vi "Engine Simulation Initialization VI.vi"(8 "error in (no error)":errorcluster, 10 "Custom XML":string, 11 "Device Item Ref in":T1 format="%.0x") -> (0 "error out":errorcluster, 3 "Device Item Ref out":T1 format="%.0x")   [LabVIEW 2011, in "Engine Sim System Explorer.lvlib"]
uses:
  Engine Sim System Explorer.lvlib
  <vilib>/NI Veristand/Custom Device API/Custom Device Item Ref.ctl
  <vilib>/NI Veristand/Custom Device API/Custom Device Loop Type.ctl
  Shared/Engine Simulation Global.vi
  <vilib>/NI Veristand/Custom Device API/Set Item Property (String).vi
  <vilib>/NI Veristand/Custom Device API/Set Item Property (Boolean).vi
  <vilib>/NI Veristand/Custom Device API/Custom Device API.lvlib
  Engine Simulation Shared.lvlib
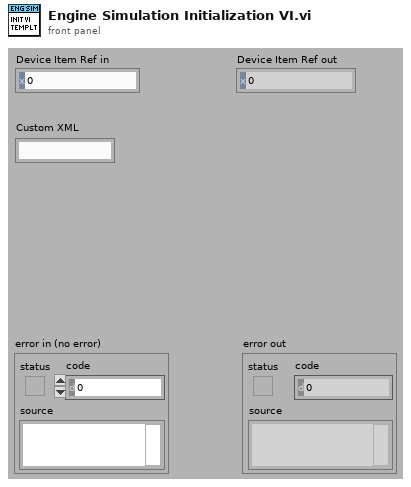
[diagram p1: front panel]
types:
  T1 = typedef "Custom Device API.lvlib/Custom Device Item Ref.ctl" = u64
  T2 = typedef "Custom Device API.lvlib/Custom Device Loop Type.ctl" = enum32{"While Loop", "Timed Loop"}
  T3 = typedef "Engine Sim System Explorer.lvlib/EngineSimComps.ctl" = cluster{"APU Component":T4, "NTeeth Components":T5[], "FullyCustom Components":T6[], "ECUEvent Components":T9[], "DataReplay Components":T10[]}
  T4 = typedef "Engine Sim System Explorer.lvlib/APUComp.ctl" = cluster{"Crank Angle":bool, "Cycle Angle":bool, "Reset":bool}
  T5 = typedef "Engine Sim System Explorer.lvlib/NTeethComp.ctl" = cluster{"Name":string, "TDC Offset":bool}
  T6 = typedef "Engine Sim System Explorer.lvlib/FullyCustomComp.ctl" = cluster{"Name":string, "Comm Mode":T7, "Profiles":T8[]}
  T7 = typedef "Engine Simulation Shared.lvlib/FullyCustomCommMode.ctl" = enum16{"DMA FIFO", "FP Data Transfer"}
  T8 = typedef "Engine Sim System Explorer.lvlib/FullyCustomProfilesComp.ctl" = cluster{"Name":string, "Offset?":bool}
  T9 = typedef "Engine Sim System Explorer.lvlib/ECUEventComp.ctl" = cluster{"Name":string, "Time Duration":bool, "Start Angle":bool, "End Angle":bool, "Angle Duration":bool}
  T10 = typedef "Engine Sim System Explorer.lvlib/DataReplayLoopComp.ctl" = cluster{"Name":string, "DataReplays":T11[]}
  T11 = typedef "Engine Sim System Explorer.lvlib/DataReplayComp.ctl" = cluster{"Name":string, "Number":i32, "Optionals":bool[]}
  T12 = cluster{"RIO Device Address":string, "Engine Sim Components":T3}
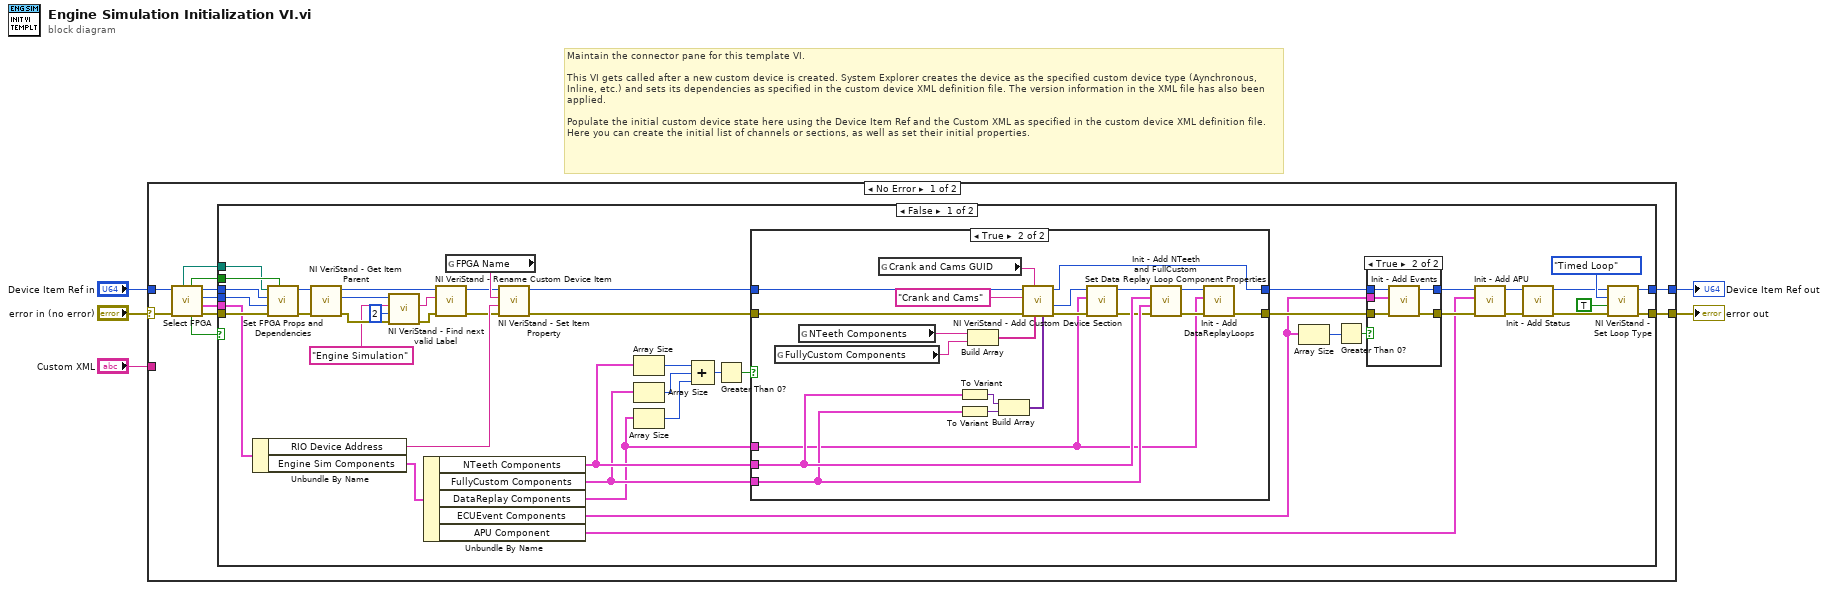
[diagram p0: block diagram]
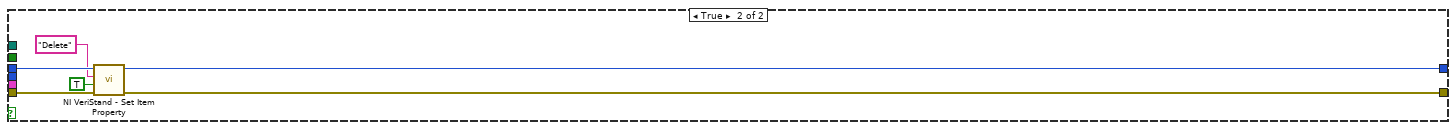
[diagram p4: hidden frame]
diagram:
  # "Maintain the connector pane for this template VI.\n\nThis VI gets called after a new custom device is created. System Explorer creates the device as the specified custom device type (Aynchronous, Inline, etc.) and sets its dependencies as specified in the custom device XML definition file. The version information in the XML file has also been applied.\n\nPopulate the initial custom device state here using the Device Item Ref and the Custom XML as specified in the custom device XML definition file. Here you can create the initial list of channels or sections, as well as set their initial properties."
  n1 = case shown="No Error" "error in (no error)" {
    selector: "error in (no error)" -> [w15 w100]
    tunnel: [w8 w100] -> w5
    tunnel: [w7 w99] -> w3
    tunnel: "Device Item Ref in" -> [w16 w99]
    tunnel: "Custom XML" -> [_ _]
    frame No Error {
      n2 = call "Select FPGA.vi"("error in"=w15, "Item Ref in"=w16) -> ("error out"=w13:errorcluster, "FPGA Info"=w11:T12, "FPGA Reference"=w14:T1, "Item Ref out"=w12:T1, "Cancelled?"=w6:bool, "VS FPGA?"=w10:bool, "Bitfile Path out"=w9:path)  [unwired: 3 in]
      n3 = case shown="False" w6 {
        tunnel: w14 -> [w59 _]
        tunnel: w13 -> [w58 w96]
        tunnel: w12 -> [w57 w98]
        tunnel: w11 -> [w56 _]
        tunnel: w10 -> [w55 _]
        tunnel: w9 -> [w54 _]
        tunnel: [w30 w95] -> w8
        tunnel: [w29 w94] -> w7
        frame False {
          n4 = Unbundle By Name(w56) -> ("RIO Device Address"=w40:string, "Engine Sim Components"=w53:T3)
          n5 = call "Set FPGA Props and Dependencies.vi"("VS FPGA?"=w55, "error in (no error)"=w58, "FPGA Ref"=w59, "CD Ref in"=w57, "Win User BF Path"=w54) -> ("error out"=w22:errorcluster, "CD Ref out"=w21:T1)  [unwired: 5 in]
          n6 = call <vilib>:"NI VeriStand - Get Item Parent.vi"("error in (no error)"=w22, "Item Ref in"=w21) -> ("error out"=w36:errorcluster, "Parent Ref"=w38:T1, "Item Ref out"=w39:T1)  [unwired: 6 in, 1 out]
          n7 = call <vilib>:"NI VeriStand - Find next valid Label.vi"("error in (no error)"=w36, "Start Value (1)"=2, "Label"="Engine Simulation", "Item Ref in"=w38) -> ("error out"=w35:errorcluster, "Label out"=w37:string)  [unwired: 3 in, 3 out]
          n8 = Unbundle By Name(w53) -> ("NTeeth Components"=w50:T5[], "FullyCustom Components"=w49:T6[], "DataReplay Components"=w17:T10[], "ECUEvent Components"=w44:T9[], "APU Component"=w52:T4)
          n9 = call <vilib>:"NI VeriStand - Rename Custom Device Item.vi"("error in (no error)"=w35, "New Name"=w37, "Item Ref in"=w39) -> ("error out"=w20:errorcluster, "Item Ref out"=w19:T1)  [unwired: 6 in, 1 out]
          n10 = global read "Engine Simulation Global.vi" "FPGA Name"() -> (w41:string)
          n11 = call-poly <vilib>:"NI VeriStand - Set Item Property.vi"("error in (no error)"=w20, "Value"=w40, "Property Name"=w41, "Item Ref in"=w19) -> ("error out"=w27:errorcluster, "Item Ref out"=w28:T1)  [unwired: 5 in, 1 out]
          n12 = Array Size(array=w50) -> (size(s)=w48:i32)
          n13 = Array Size(array=w49) -> (size(s)=w47:i32)
          n14 = Array Size(array=w17) -> (size(s)=w18:i32)
          n15 = Compound Arithmetic op=ADD(w48, w47, w18) -> (w46:i32)
          n16 = Greater Than 0?(x=w46) -> (x > 0?=w45:bool)
          n17 = case shown="True" w45 {
            tunnel: [w70 w79] -> w62
            tunnel: w27 -> [w71 w86]
            tunnel: w28 -> [w70 w85]
            tunnel: w50 -> [_ w81]
            tunnel: [w71 w77] -> w51
            tunnel: w49 -> [_ w80]
            tunnel: w17 -> [_ w72]
            frame False {
            }
            frame True {
              n18 = global read "Engine Simulation Global.vi" "FullyCustom Components"() -> (w91:string)
              n19 = global read "Engine Simulation Global.vi" "NTeeth Components"() -> (w89:string)
              n20 = global read "Engine Simulation Global.vi" "Crank and Cams GUID"() -> (w87:string)
              n21 = To Variant(anything=w81) -> (Variant=w83:variant)
              n22 = To Variant(anything=w80) -> (Variant=w84:variant)
              n23 = Build Array(w89, w91) -> (w90:string[])
              n24 = Build Array(w83, w84) -> (w82:variant[])
              n25 = call <vilib>:"NI VeriStand - Add Custom Device Section.vi"("Property Values"=w82, "Property names"=w90, "GUID (Default Section)"=w87, "error in (no error)"=w86, "Section Name"="Crank and Cams", "Parent Ref in"=w85) -> ("error out"=w78:errorcluster, "Section Ptr"=w74:T1, "Parent Ref out"=w79:T1)  [unwired: 2 in, 1 out]
              n26 = call "Set Data Replay Loop Component Properties.vi"("error in (no error)"=w78, "DataReplayLoops"=w72, "Item Ref in"=w74) -> ("error out"=w75:errorcluster, "Item Ref out"=w73:T1)  [unwired: 7 in]
              n27 = call "Init - Add NTeeth and FullCustom.vi"("error in (no error)"=w75, "FullyCustom Components"=w80, "NTeeth Components"=w81, "Crank Cams Page in"=w73) -> ("error out"=w92:errorcluster, "Crank Cams Page out"=w76:T1)  [unwired: 6 in]
              n28 = call "Init - Add DataReplayLoops.vi"("error in (no error)"=w92, "DataReplay Components"=w72, "Crank Cams Page in"=w76) -> ("error out"=w77:errorcluster)  [unwired: 7 in, 1 out]
            }
          }
          n29 = Array Size(array=w44) -> (size(s)=w43:i32)
          n30 = Greater Than 0?(x=w43) -> (x > 0?=w42:bool)
          n31 = case shown="True" w42 {
            tunnel: w62 -> [w64 w69]
            tunnel: [w64 w68] -> w61
            tunnel: [w63 w65] -> w60
            tunnel: w51 -> [w63 w67]
            tunnel: w44 -> [_ w66]
            frame False {
            }
            frame True {
              n32 = call "Init - Add Events.vi"("error in (no error)"=w67, "ECUEvent Components"=w66, "Device ref in"=w69) -> ("error out"=w65:errorcluster, "Device ref out"=w68:T1)  [unwired: 7 in]
            }
          }
          n33 = call "Init - Add APU.vi"("error in (no error)"=w60, "APU Component"=w52, "Device ref in"=w61) -> ("error out"=w26:errorcluster, "Device Ref out"=w25:T1)  [unwired: 7 in]
          n34 = call "Init - Add Status.vi"("error in (no error)"=w26, "Device Ref in"=w25) -> ("error out"=w23:errorcluster, "Parent Ref out"=w24:T1)  [unwired: 8 in]
          n35 = call <vilib>:"NI VeriStand - Set Loop Type.vi"("error in (no error)"=w23, "Use Device Clock (Timed Loops only)"=TRUE, "Loop type"=Custom_Device_Loop_Type."Timed Loop", "Device Ref in"=w24) -> ("error out"=w30:errorcluster, "Device Ref out"=w29:T1)  [unwired: 6 in]
        }
        frame True {
          n36 = call-poly <vilib>:"NI VeriStand - Set Item Property.vi"("error in (no error)"=w96, "Value"=TRUE ("Force Delete (F)"), "Property Name"="Delete", "Item Ref in"=w98) -> ("error out"=w95:errorcluster, "Item Ref out"=w94:T1)  [unwired: 5 in, 1 out]
        }
      }
    }
    frame Error {
    }
  }
  "error out" <- w5
  "Device Item Ref out" <- w3
